vi "SanityCheck.vi"() -> ()   [LabVIEW 2014]
uses:
  <vilib>/addons/h5labview2/file/H5Fmode.ctl
  <vilib>/addons/h5labview2/base/lib_path.vi
  <vilib>/addons/h5labview2/base/H5Equery.vi
  <vilib>/addons/h5labview2/dataset/H5Dwrite.llb/H5Dwrite.xnode
  <vilib>/addons/h5labview2/file/H5F.lvlib
  <vilib>/addons/h5labview2/group/H5G.lvlib
  <vilib>/addons/h5labview2/attrib/H5A.lvlib
panel:
  in  "path":path
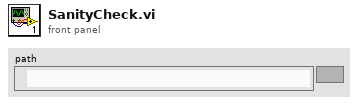
[diagram p1: front panel]
types:
  T1 = typedef "H5F.lvlib/H5Fmode.ctl" = enum16{"read-only", "read-write", "overwrite", "create new", "open or create"}
  T2 = typedef "hid_t.ctl" = i32
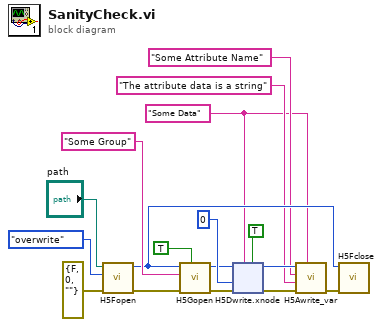
[diagram p0: block diagram]
diagram:
  w2 = "Some Data" ("name")
  n1 = call <vilib>:"H5Fopen.vi"("error in (no error)"=errorcluster {"status"=FALSE, "code"=0, "source"=""}, "mode (read-only)"=H5Fmode."overwrite", "path"="path") -> ("error out"=w14:errorcluster, "ref out"=w12:T2)  [unwired: 7 in]
  n2 = call <vilib>:"H5Gopen.vi"("create? (F)"=TRUE, "error in (no error)"=w14, "name"="Some Group", "ref in"=w12) -> ("error out"=w5:errorcluster, "group out"=w3:T2)  [unwired: 6 in]
  n3 = xnode "H5Dwrite.xnode"("replace? (F)"=TRUE, "dataset name"=w2, "error in (no error)"=w5, "data"=0, "ref in"=w3) -> ("error out"=w7:errorcluster, "ref out"=w10:i32)  [unwired: 2 in, 1 out]
  n4 = call <vilib>:"H5Awrite_var.vi"("object name"=w2, "error in (no error)"=w7, "data"="The attribute data is a string", "attrib name"="Some Attribute Name", "ref in"=w10) -> ("error out"=w6:errorcluster)  [unwired: 4 in, 2 out]
  n5 = call <vilib>:"H5Fclose.vi"("error in (no error)"=w6, "ref"=w12) -> ()  [unwired: 9 in, 1 out]
